vi "Microscope.SetConfiguration.vi"(8 "error in (no error)":errorcluster, 10 "Configuration":T1={"XY Stage"="", "Camera"="", "image output folder"=path "", "filetype"="png"}, 11 "Microscope":refnum<class "Microscope.lvclass">) -> (0 "error out":errorcluster, 3 "Microscope out":refnum<class "Microscope.lvclass">)   [LabVIEW 2013, in "Microscope.lvclass"]
doc: "---------------------------------------------------------------\nJKI State Machine Objects™\nhttp://jki.net/state-machine-objects/\nCopyright (C) 2005-2015, JKI <info@jki.net>\nALL RIGHTS RESERVEDJKI State Machine Objects (SMO) 1.0.0.5\nJKI - JKI\nCopyright (c) 2016, JKI"
uses:
  Microscope.lvclass
  Typedefs/Configuration--Cluster.ctl
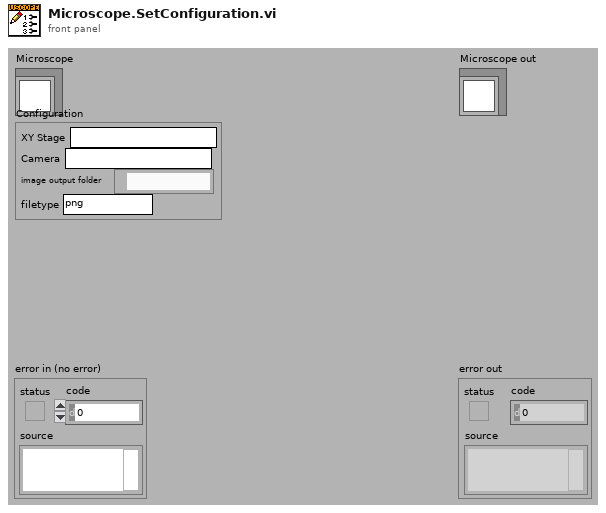
[diagram p1: front panel]
types:
  T1 = typedef "Microscope.lvclass/Configuration--Cluster.ctl" = cluster{"XY Stage":string, "Camera":string, "image output folder":path, "filetype":string}
  T2 = typedef "Microscope.lvclass/PrivateData--Ref.ctl" = refnum<data-value>
  T3 = typedef "Microscope.lvclass/PrivateData--Cluster.ctl" = cluster{"Public Events":T4, "Protected Events":T5, "Private Events":T6, "Dependencies":T7, "Configuration":T1}
  T4 = typedef "Microscope.lvclass/PublicEvents--Cluster.ctl" = cluster{"Value Changed":refnum<user-event>, "Initialized":refnum<user-event>}
  T5 = typedef "Microscope.lvclass/ProtectedEvents--Cluster.ctl" = cluster{"placeholder":refnum<user-event>}
  T6 = typedef "Microscope.lvclass/PrivateEvents--Cluster.ctl" = cluster{"New Value":refnum<user-event>, "Initialize":refnum<user-event>, "CaptureImageAtPosition":refnum<user-event>}
  T7 = typedef "Microscope.lvclass/Dependencies--Cluster.ctl" = cluster{"XYStage":refnum<class "XYStage.lvclass">, "Camera":refnum<class "Camera.lvclass">}
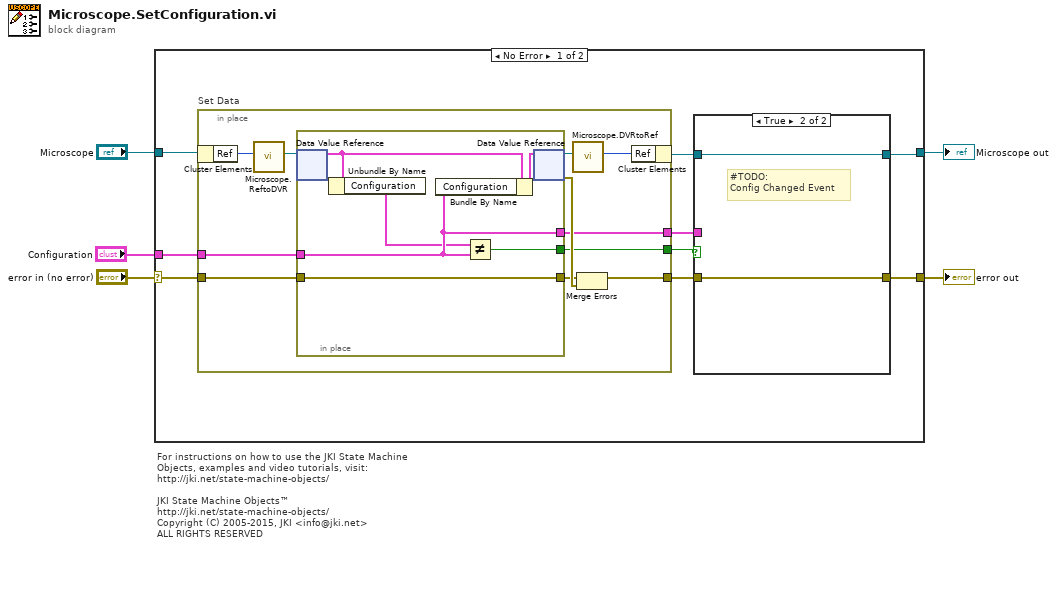
[diagram p0: block diagram]
diagram:
  # "For instructions on how to use the JKI State Machine Objects, examples and video tutorials, visit:\nhttp://jki.net/state-machine-objects/\n\nJKI State Machine Objects™\nhttp://jki.net/state-machine-objects/\nCopyright (C) 2005-2015, JKI <info@jki.net>\nALL RIGHTS RESERVED"
  n1 = case shown="No Error" "error in (no error)" {
    selector: "error in (no error)" -> [w13 w36]
    tunnel: "Microscope" -> [w14 w37]
    tunnel: [w7 w36] -> w5
    tunnel: [w8 w37] -> w4
    tunnel: "Configuration" -> [w12 _]
    frame No Error {
      n2 = in-place "Set Data" {
        in-place-border: w13 -> [w29]
        in-place-border: [w26] -> w6
        in-place-border: w12 -> [w19]
        in-place-border: [w25] -> w10
        in-place-border: [w20] -> w11
        n3 = in-place-cluster #1(w14) -> ("Ref"=w24:u32)
        n4 = call "Microscope.ReftoDVR.vi"("Ref"=w24) -> ("Ref"=w23:T2)  [unwired: 10 in]
        n5 = in-place {
          in-place-border: w29 -> [w35]
          in-place-border: [w35] -> w27
          in-place-border: w19 -> [w32]
          in-place-border: [w32] -> w25
          in-place-border: [w30] -> w20
          n6 = in-place-dvr #2(w23) -> (w33:T3)  [unwired: 1 out]
          n7 = Unbundle By Name(w33) -> ("Configuration"=w31:T1)
          n8 = Bundle By Name(cluster=w33, "Configuration"=w32) -> (w34:T3)
          n9 = Not Equal?(x=w31, y=w32) -> (x != y?=w30:bool)
          n10 = in-place-dvr #2(w34) -> (w22:T2, w28:errorcluster)
        }
        n11 = call "Microscope.DVRtoRef.vi"("Ref"=w22) -> ("Ref"=w21:u32)  [unwired: 10 in]
        n12 = Merge Errors(w27, w28) -> (w26:errorcluster)
        n13 = in-place-cluster #1("Ref"=w21) -> (w9:refnum<class "Microscope.lvclass">)
      }
      n14 = case shown="True" w11 {
        tunnel: w10 -> [_ _]
        tunnel: w9 -> [w16 w18]
        tunnel: [w16 w18] -> w8
        tunnel: w6 -> [w15 w17]
        tunnel: [w15 w17] -> w7
        frame False {
        }
        frame True {
          # "#TODO: \nConfig Changed Event"
        }
      }
    }
    frame Error {
      # "Upstream error or State Machine Object has not been created."
    }
  }
  "error out" <- w5
  "Microscope out" <- w4
